vi "Create Mesh.vi"(7 "3D Surface Property":T4={"General Property"={"Plot Name"="", "Coordinate System"=enum."Cartesian", "Opacity"=0.0}, "Projection Property"={"Draw XY"=FALSE, "Draw YZ"=FALSE, "Draw XZ"=FALSE}, "Plot Property"={"Draw Surface"=FALSE, "Draw Mesh"=FALSE, "Draw Normal"=FALSE, "Color Ramp Cluster"={"Color Ramp Style"=enum."None", "Color Ramp Array"=[16711934, 393471, 57855, 4390754, 16449346, 16744722, 16711680], "Color Ramp Index"=[45, 91, 133, 175, 219, 255], "Interpolate?"=FALSE, "Logarithm?"=FALSE}, "Line Style"=enum."None", "Line Width"=0.0, "Line Color"=0, "Antialiasing"=FALSE}, "Surface Property"={"Color Mode"=enum."Flat Shading"}}, 8 "error in (no error)":errorcluster, 9 "Actual Transform In":T7, 10 "Plot Representation In":T1, 11 "Plot Object In":refnum<vi>) -> (0 "error out":errorcluster, 1 "Actual Transform Out":T7, 2 "Plot Representation Out":T1, 3 "Plot Object Out":refnum<vi>, 4 "Mesh Object Out":refnum<vi>)   [LabVIEW 2020, in "3D Surface.lvclass"]
uses:
  3D Surface.lvclass
  Actual Transform.ctl
  Range Clusters.ctl
  Plot Representation.ctl
  Mesh Data.ctl
  3D Surface Property.ctl
  Color Ramp Cluster.ctl
  Line Type.ctl
  NI_3D Picture Control.lvlib
  3D Plot.lvclass
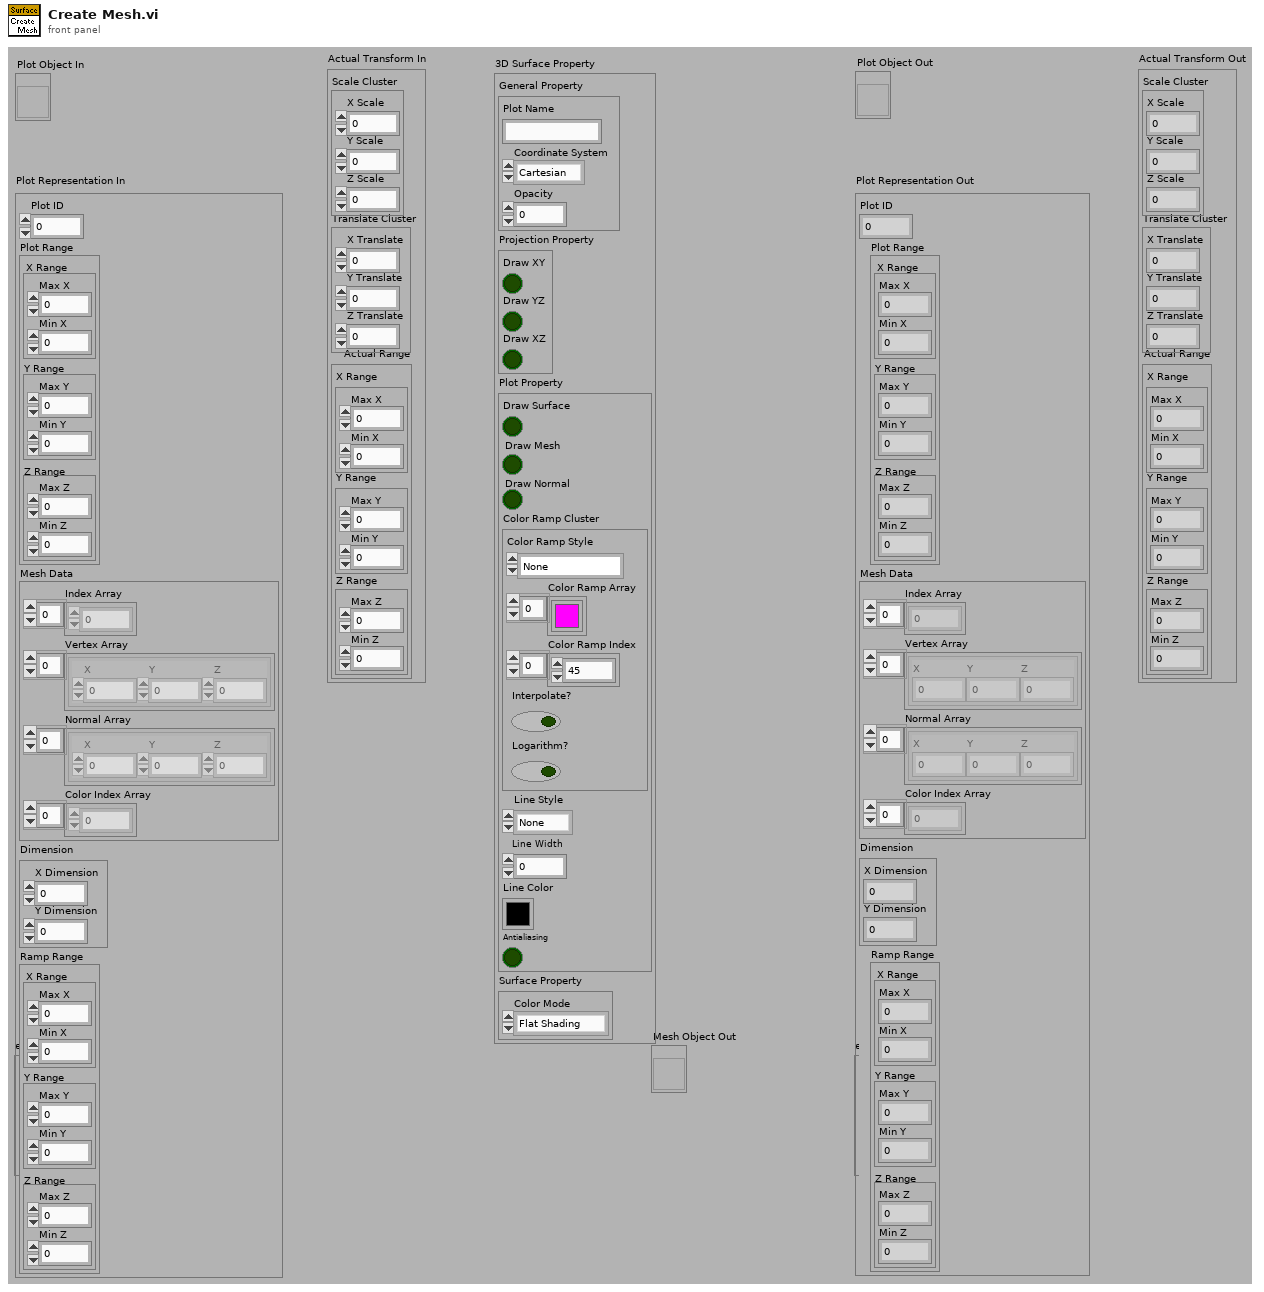
[diagram p1: front panel]
types:
  T1 = typedef "3D Plot.lvclass/Plot Representation.ctl" = cluster{"Plot ID":i32, "Plot Range":T2, "Mesh Data":T3, "Dimension":cluster{"X Dimension":i32, "Y Dimension":i32}, "Ramp Range":T2}
  T2 = typedef "3D Plot.lvclass/Range Clusters.ctl" = cluster{"X Range":cluster{"Max X":sgl, "Min X":sgl}, "Y Range":cluster{"Max Y":sgl, "Min Y":sgl}, "Z Range":cluster{"Max Z":sgl, "Min Z":sgl}}
  T3 = typedef "3D Plot.lvclass/Mesh Data.ctl" = cluster{"Index Array":u32[], "Vertex Array":cluster{"X":sgl, "Y":sgl, "Z":sgl}[], "Normal Array":cluster{"X":sgl, "Y":sgl, "Z":sgl}[], "Color Index Array":i32[]}
  T4 = typedef "3D Surface.lvclass/3D Surface Property.ctl" = cluster{"General Property":cluster{"Plot Name":string, "Coordinate System":enum16{"Cartesian", "Cylindrical", "Spherical"}, "Opacity":sgl}, "Projection Property":cluster{"Draw XY":bool, "Draw YZ":bool, "Draw XZ":bool}, "Plot Property":cluster{"Draw Surface":bool, "Draw Mesh":bool, "Draw Normal":bool, "Color Ramp Cluster":T5, "Line Style":T6, "Line Width":sgl, "Line Color":u32, "Antialiasing":bool}, "Surface Property":cluster{"Color Mode":enum16{"Flat Shading", "Interpolated Shading"}}}
  T5 = typedef "3D Plot.lvclass/Color Ramp Cluster.ctl" = cluster{"Color Ramp Style":enum16{"None", "Shaded", "Color spectrum", "Grey scale", "Custom"}, "Color Ramp Array":u32[], "Color Ramp Index":i32[], "Interpolate?":bool, "Logarithm?":bool}
  T6 = typedef "3D Plot.lvclass/Line Type.ctl" = enum16{"None", "Solid", "Dash", "Dot", "Dash Dot"}
  T7 = typedef "3D Plot.lvclass/Actual Transform.ctl" = cluster{"Scale Cluster":cluster{"X Scale":sgl, "Y Scale":sgl, "Z Scale":sgl}, "Translate Cluster":cluster{"X Translate":sgl, "Y Translate":sgl, "Z Translate":sgl}, "Actual Range":T2}
  T8 = enum16{"Points", "Lines", "Line Strip", "Line Loop", "Triangles", "Triangle Strip", "Triangle Fan", "Quads", "Quad Strip", "Polygon"}
  T9 = enum16{"Overall", "Per Primitive", "Per Vertex", "Binding Off"}
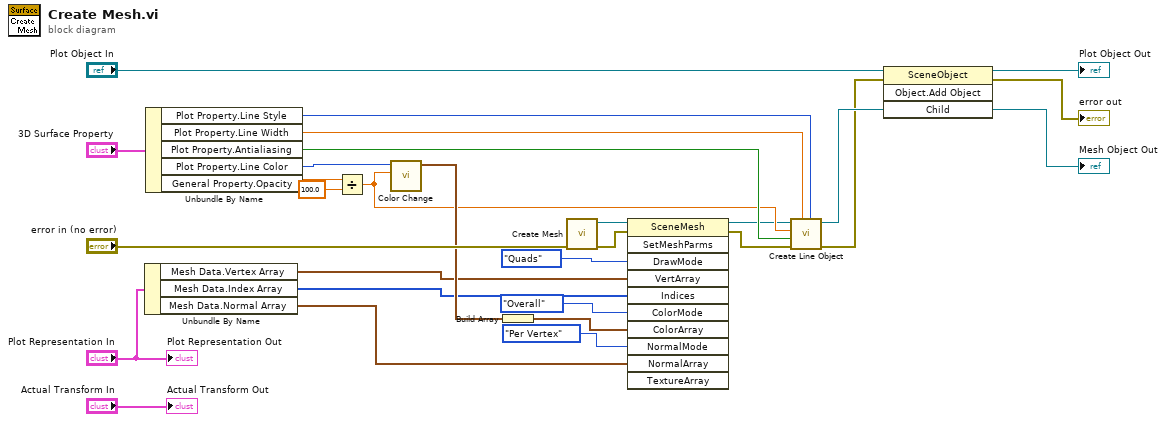
[diagram p0: block diagram]
diagram:
  n1 = Unbundle By Name("Plot Representation In") -> ("Mesh Data.Vertex Array"=w17:cluster{"X":sgl, "Y":sgl, "Z":sgl}[], "Mesh Data.Index Array"=w16:u32[], "Mesh Data.Normal Array"=w21:cluster{"X":sgl, "Y":sgl, "Z":sgl}[])
  n2 = Unbundle By Name("3D Surface Property") -> ("Plot Property.Line Style"=w12:T6, "Plot Property.Line Width"=w15:sgl, "Plot Property.Antialiasing"=w13:bool, "Plot Property.Line Color"=w20:u32, "General Property.Opacity"=w14:sgl)
  n3 = Divide(x=w14, y=sgl 100.0) -> (x/y=w11:sgl)
  n4 = call "Color Change.vi"("Alpha"=w11, "Color"=w20) -> ("RGBA"=w19:cluster{"R":sgl, "G":sgl, "B":sgl, "A":sgl})  [unwired: 9 out]
  n5 = Build Array(w19) -> (w4:cluster{"R":sgl, "G":sgl, "B":sgl, "A":sgl}[])
  n6 = call "Create Mesh.vi"("error in (no error)"="error in (no error)") -> ("error out"=w7:errorcluster, "New Mesh Refnum"=w10:refnum<vi>)  [unwired: 9 out]
  n7 = invoke class="SceneMesh" method="SetMeshParms"(reference=w10, error in=w7, "DrawMode"=T8."Quads" ("Draw Mode"), "VertArray"=w17, "Indices"=w16, "ColorMode"=T9."Overall" ("Color Binding Mode"), "ColorArray"=w4, "NormalMode"=T9."Per Vertex" ("Normal Binding Mode"), "NormalArray"=w21) -> (reference out=w9:refnum<vi>, error out=w6:errorcluster)  [unwired: 2 in, 9 out]
  n8 = call "Create Line Object.vi"("Line Style"=w12, "Line Width"=w15, "error in (no error)"=w6, "Antialiasing"=w13, "Alpha"=w11, "Mesh Ref In"=w9) -> ("error out"=w2:errorcluster, "Object Ref Out"=w5:refnum<vi>)  [unwired: 4 out]
  n9 = invoke class="SceneObject" method="Object.Add Object"(reference="Plot Object In", error in=w2, "Child"=w5) -> (reference out=→"Plot Object Out":refnum<vi>, error out=→"error out":errorcluster, "Child"=→"Mesh Object Out":refnum<vi>)  [unwired: 1 in, 1 out]
  "Actual Transform Out" <- "Actual Transform In"
  "Plot Representation Out" <- "Plot Representation In"
